vi "GEOM_CleanROIs.vi"(9 "Binning":T1={"x"=1, "y"=1} {"y" min=1; "x" min=1}, 10 "amplifiers in":T2[](array[typedef]) {"fliped" items=["none", "horizontal", "vertical"]; "type" items=["LL", "LR", "UL", "UR"]}) -> (2 "amplifiers out":T2[](array[typedef]) {"fliped" items=["none", "horizontal", "vertical"]; "type" items=["LL", "LR", "UL", "UR"]})   [LabVIEW 2016]
uses:
  GEOM_Amplifier.ctl
  GEOM_AmpType.ctl
  GEOM_ROI.ctl
  GEOM_Coords.ctl
  GEOM_Binning.ctl
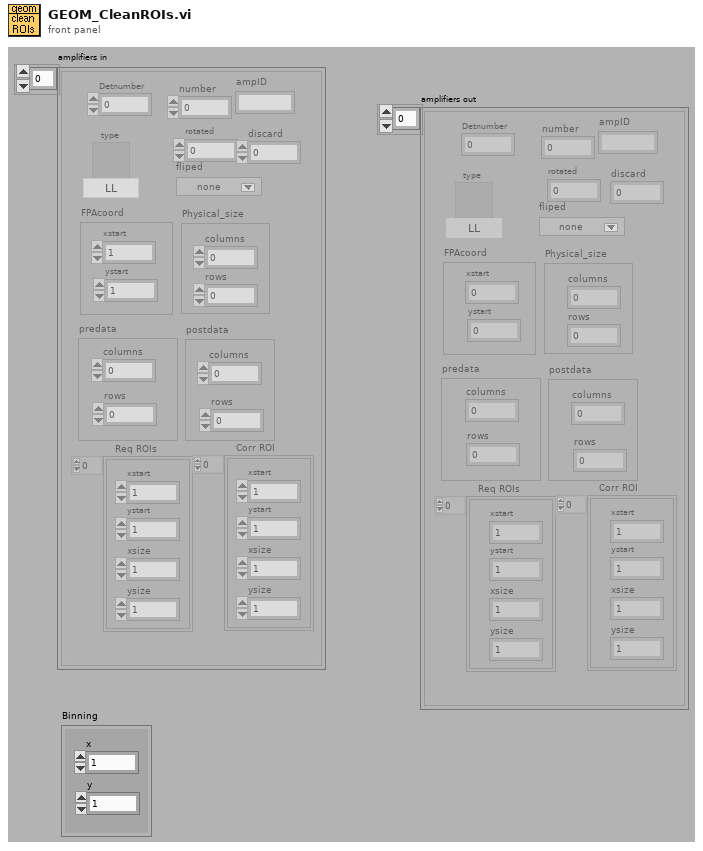
[diagram p1: front panel]
types:
  T1 = typedef "GEOM_Binning.ctl" = cluster{"x":u32, "y":u32}
  T2 = typedef "GEOM_Amplifier.ctl" = cluster{"number":i32, "type":T3, "rotated":i16, "fliped":u16, "FPAcoord":cluster{"xstart":i32, "ystart":i32}, "Physical_size":cluster{"columns":i32, "rows":i32}, "predata":cluster{"columns":i32, "rows":i32}, "postdata":cluster{"columns":i32, "rows":i32}, "Req ROIs":T4, "Corr ROI":T4, "Detnumber":i32, "ampID":string, "discard":i32}
  T3 = typedef "GEOM_AmpType.ctl" = u16
  T4 = typedef "GEOM_ROI.ctl" = T5[]
  T5 = typedef "GEOM_Coords.ctl" = cluster{"xstart":u32, "ystart":u32, "xsize":u32, "ysize":u32}
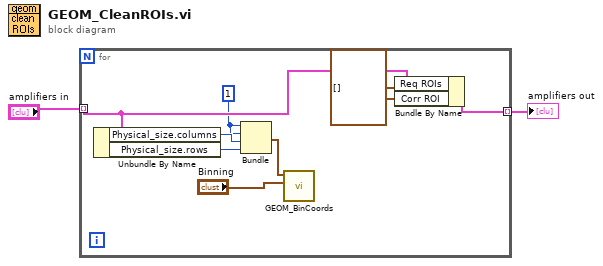
[diagram p0: block diagram]
diagram:
  n1 = for {
    tunnel: "amplifiers in" -> [w8] mode=indexing
    tunnel: [w10] -> w2 mode=indexing
    w3 = T4 [] ("Req ROIs")
    w5 = 1
    n2 = Unbundle By Name(w8) -> ("Physical_size.columns"=w6:i32, "Physical_size.rows"=w7:i32)
    n3 = Bundle(w5, w5, "columns"=w6, "rows"=w7) -> (w4:cluster{i32, i32, "columns":i32, "rows":i32})  [unwired: 1 out]
    n4 = call "GEOM_BinCoords.vi"("Binning"="Binning", "coords"=w4) -> ()  [unwired: 2 in, 8 out]
    n5 = Bundle By Name(cluster=w8, "Req ROIs"=w3, "Corr ROI"=w3) -> (w10:T2)
  }
  "amplifiers out" <- w2
